vi "Status TimerOn.vi"(8 "error in (no error)":errorcluster, 10 "Address (0)":i32, 11 "VISA resource name":refnum<visa-resource-name>) -> (0 "error out":errorcluster, 1 "Timer Numbers":T1[](array[typedef]), 2 "Valid Timers":i32, 3 "VISA resource name out":refnum<visa-resource-name>)   [LabVIEW 2016, in "Environment Chamber.lvlib" / "Climatic Chamber.lvlib"]
doc: "<b>Active timer monitor</b>\n\nReturns the number of active timers and the timer numbers."
uses:
  Climatic Chamber.lvlib
  Private/Type Defs/TimerNumber Enum.ctl
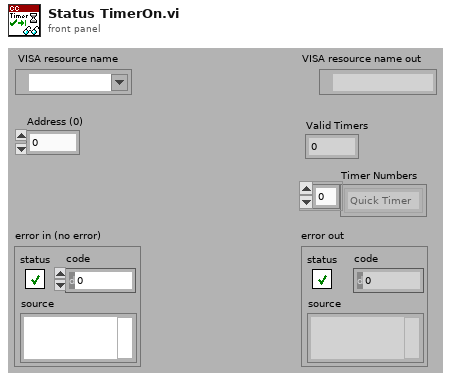
[diagram p1: front panel]
types:
  T1 = typedef "Environment Chamber.lvlib/Climatic Chamber.lvlib/TimerNumber Enum.ctl" = enum16{"Quick Timer", "Start Timer", "End Timer"}
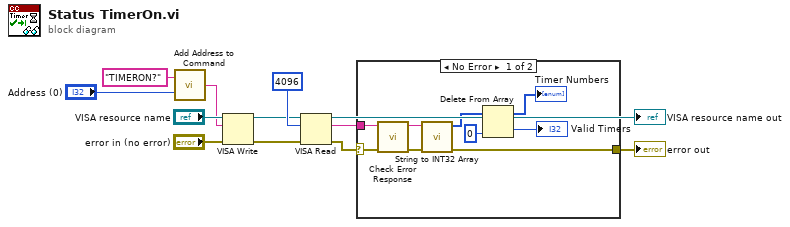
[diagram p0: block diagram]
diagram:
  n1 = call "Add Address to Command.vi"("Address (0)"="Address (0)", "Command"="TIMERON?") -> ("Command OUT"=w5:string)
  n2 = VISA Write(VISA resource name="VISA resource name", write buffer=w5, error in (no error)="error in (no error)") -> (VISA resource name out=w9:refnum<visa-resource-name>, error out=w8:errorcluster)  [unwired: 1 out]
  n3 = VISA Read(VISA resource name=w9, byte count=u32 4096, error in (no error)=w8) -> (VISA resource name out=→"VISA resource name out":refnum<visa-resource-name>, read buffer=w3:string, error out=w4:errorcluster)  [unwired: 1 out]
  n4 = case shown="No Error" w4 {
    selector: w4 -> [w20 w22]
    tunnel: w3 -> [w21 _]
    tunnel: [w18 w22] -> w2
    frame No Error {
      n5 = call "Check Error Response.vi"("error in (no error)"=w20, "read String"=w21) -> ("error out"=w19:errorcluster, "String out"=w17:string)  [unwired: 7 in, 1 out]
      n6 = call "String to INT32 Array.vi"("error in (no error)"=w19, "String received"=w17) -> ("error out"=w18:errorcluster, "Array Data"=w16:i32[])  [unwired: 8 in]
      n7 = Delete From Array(array=w16, index=0) -> (deleted portion=→"Valid Timers":i32, array with subset deleted=→"Timer Numbers":i32[])  [unwired: 1 in]
    }
    frame Error {
    }
  }
  "error out" <- w2
